vi "SaveMaskList.vi"(7 "dxfFile":string, 8 "UiDefinition 2":T1, 9 "url":string, 10 "Masks":string, 11 ".NET Refnum in":refnum<k24>) -> ()   [LabVIEW 2020]
uses:
  D:/LabviewDXFViewer/LabviewDXFViewer/bin/Release/LabviewDXFViewer.exe
  LabviewDXFViewer/bin/Release/LabviewDXFViewer.exe
  UIReferences.ctl
  <vilib>/httpClient/POSTBuffer.vi
  <vilib>/httpClient/LabVIEWHTTPClient.lvlib
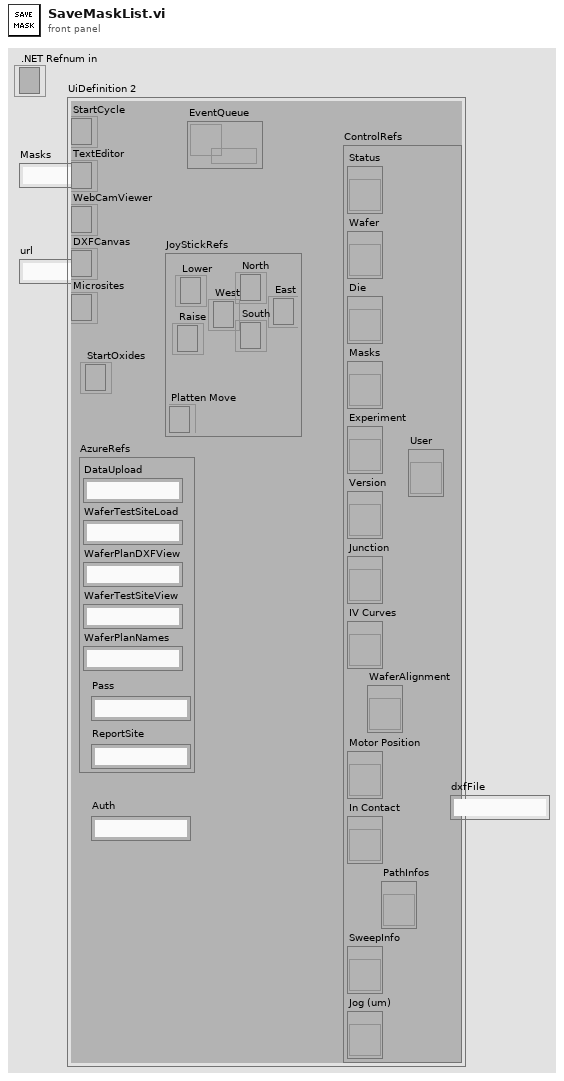
[diagram p1: front panel]
types:
  T1 = typedef "UIReferences.ctl" = cluster{"StartCycle":refnum<k24>, "TextEditor":refnum<k24>, "WebCamViewer":refnum<k24>, "DXFCanvas":refnum<k24>, "Microsites":refnum<k24>, "JoyStickRefs":cluster{"North":refnum<k24>, "Lower":refnum<k24>, "Raise":refnum<k24>, "Platten Move":refnum<k24>, "West":refnum<k24>, "East":refnum<k24>, "South":refnum<k24>}, "AzureRefs":cluster{"DataUpload":string, "WaferTestSiteLoad":string, "WaferPlanDXFView":string, "WaferTestSiteView":string, "WaferPlanNames":string, "Pass":string, "ReportSite":string}, "ControlRefs":cluster{"Status":refnum<vi>, "Wafer":refnum<vi>, "Die":refnum<vi>, "Masks":refnum<vi>, "Experiment":refnum<vi>, "Version":refnum<vi>, "Junction":refnum<vi>, "IV Curves":refnum<vi>, "Motor Position":refnum<vi>, "In Contact":refnum<vi>, "SweepInfo":refnum<vi>, "Jog (um)":refnum<vi>, "PathInfos":refnum<vi>, "User":refnum<vi>, "WaferAlignment":refnum<vi>}, "EventQueue":refnum<queue>, "StartOxides":refnum<k24>, "Auth":string}
  T2 = typedef "LabVIEWHTTPClient.lvlib/ClientHandle.ctl" = refnum<k1>
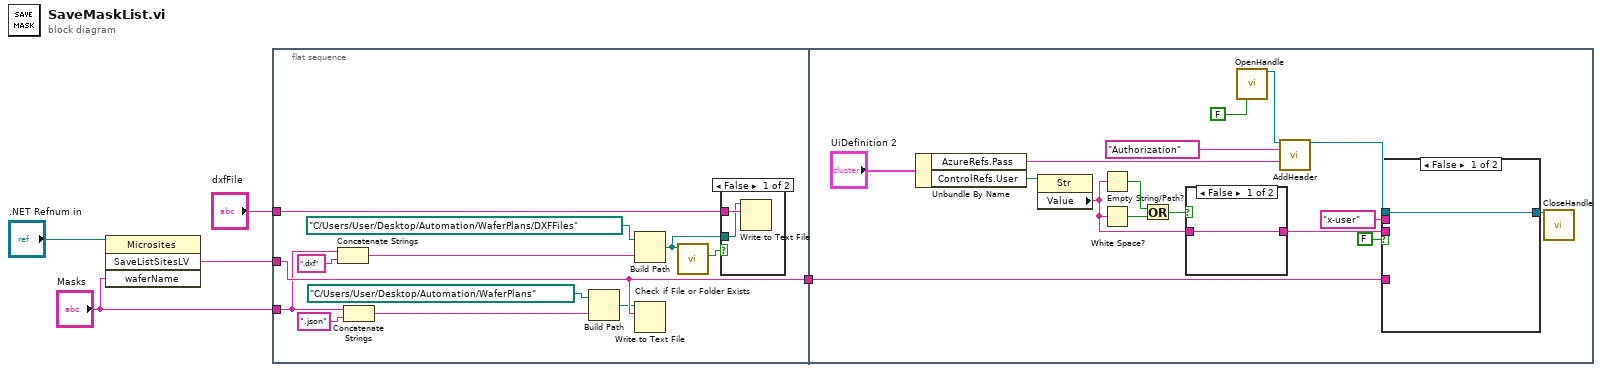
[diagram p0: block diagram]
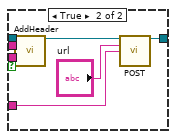
[diagram p3: hidden frame]
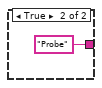
[diagram p4: hidden frame]
diagram:
  n1 = invoke class="Microsites" method="SaveListSitesLV"(reference=".NET Refnum in", "waferName"="Masks") -> ("SaveListSitesLV"=w4:string)  [unwired: 2 in, 3 out]
  n2 = flat-sequence {
    tunnel: w4 -> [w17]
    tunnel: [w17] -> w3
    tunnel: "Masks" -> [w9]
    tunnel: "dxfFile" -> [w8]
    tunnel: w3 -> [w21]
    frame #0 {
      n3 = Concatenate Strings(w9, ".dxf" ("string")) -> (w14:string)
      n4 = Concatenate Strings(w9, ".json" ("string")) -> (w11:string)
      n5 = Build Path(base path=path "C:/Users/User/Desktop/Automation/WaferPlans" ("file (use dialog)"), name or relative path=w11) -> (appended path=w10:path)
      n6 = Build Path(base path=path "C:/Users/User/Desktop/Automation/WaferPlans/DXFFiles" ("file (use dialog)"), name or relative path=w14) -> (appended path=w7:path)
      n7 = Write to Text File(file (use dialog)=w10, text=w17) -> ()  [unwired: 2 in, 3 out]
      n8 = call <vilib>:"Check if File or Folder Exists.vi"("path"=w7) -> ("file or folder exists?"=w6:bool)  [unwired: 8 in, 2 out]
      n9 = case shown="False" w6 {
        tunnel: w8 -> [w19 _]
        tunnel: w7 -> [w18 _]
        frame False {
          n10 = Write to Text File(file (use dialog)=w18, text=w19) -> ()  [unwired: 2 in, 3 out]
        }
        frame True {
        }
      }
    }
    frame #1 {
      n11 = Unbundle By Name("UiDefinition 2") -> ("AzureRefs.Pass"=w31:string, "ControlRefs.User"=w29:refnum<vi>)
      n12 = property class="Str"(reference=w29) -> ("Value"=w24:string)  [unwired: 1 in, 2 out]
      n13 = Empty String/Path?(string/path=w24) -> (empty?=w25:bool)
      n14 = White Space?(1:w24) -> (0:w28:bool)
      n15 = Or(x=w25, y=w28) -> (x .or. y?=w26:bool)
      n16 = case shown="False" w26 {
        tunnel: w24 -> [w44 _]
        tunnel: [w44 "Probe"] -> w27
        frame False {
        }
        frame True {
        }
      }
      n17 = call <vilib>:"OpenHandle.vi"("verify server(true)"=FALSE) -> ("client handle out"=w23:T2)  [unwired: 13 in, 1 out]
      n18 = call <vilib>:"AddHeader.vi"("client handle"=w23, "header"="Authorization", "value"=w31) -> ("client handle out"=w33:T2)  [unwired: 11 in, 1 out]
      n19 = case shown="False" FALSE {
        tunnel: [w36 w42] -> w35
        tunnel: w33 -> [w36 w41]
        tunnel: "x-user" ("header") -> [_ w40]
        tunnel: w27 -> [_ w39]
        tunnel: w21 -> [_ w37]
        frame False {
        }
        frame True {
          n20 = call <vilib>:"AddHeader.vi"("client handle"=w41, "header"=w40, "value"=w39) -> ("client handle out"=w38:T2)  [unwired: 11 in, 1 out]
          n21 = call-poly <vilib>:"POST.vi"("client handle"=w38, "url"="url", "buffer"=w37) -> ("client handle out"=w42:T2)  [unwired: 9 in, 3 out]
        }
      }
      n22 = call <vilib>:"CloseHandle.vi"("client handle"=w35) -> ()  [unwired: 14 in, 1 out]
    }
  }
